vi "Move Middle Pane Items.vi"(8 "error in":errorcluster, 10 "Vertical Distance to Move":dbl, 11 "Object References":refnum<vi>[](array[refnum])) -> (0 "error out":errorcluster)   [LabVIEW 2014]
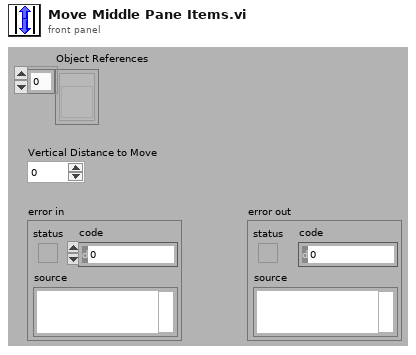
[diagram p1: front panel]
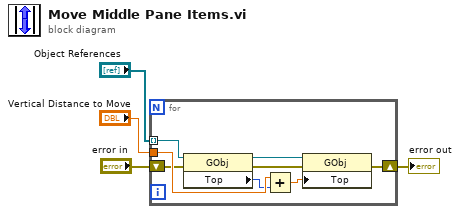
[diagram p0: block diagram]
diagram:
  n1 = for {
    tunnel: "Vertical Distance to Move" -> [w12]
    shift-right: [w11] -> w3
    shift-left: "error in" -> [w10]
    tunnel: "Object References" -> [w5] mode=indexing
    n2 = property class="GObj"(reference=w5, error in=w10) -> (reference out=w7:refnum<vi>, error out=w9:errorcluster, "Top"=w8:i32)
    n3 = Add(x=w12, y=w8) -> (x+y=w6:dbl)
    n4 = property class="GObj"(reference=w7, error in=w9, "Top"=w6) -> (error out=w11:errorcluster)  [unwired: 1 out]
  }
  "error out" <- w3
